vi "Collector Lift Manual Override.vi"(9 "Output":dbl, 10 "Collector Lift Man.  Request?":bool, 11 "Collector Lift Man. Value":dbl) -> (3 "Collector Lift Output":dbl)   [LabVIEW 2015]
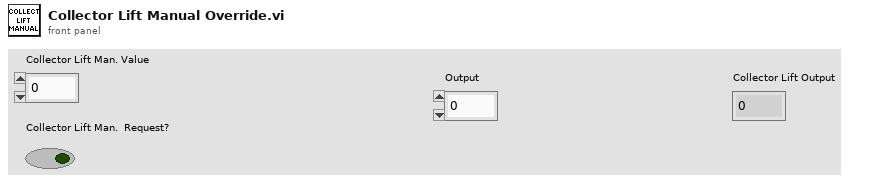
[diagram p1: front panel]
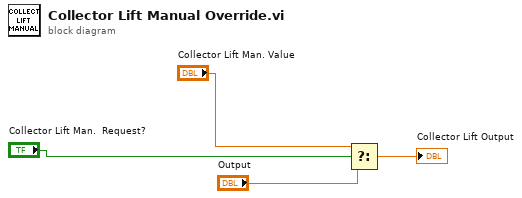
[diagram p0: block diagram]
diagram:
  n1 = Select(t="Collector Lift Man. Value", s="Collector Lift Man.  Request?", f="Output") -> (s? t:f=→"Collector Lift Output":dbl)
